vi "Write.Data.vi"(8 "error in (no error)":errorcluster, 10 "Values":dbl[](array[numeric]), 11 "Ref":refnum<data-value>) -> (0 "error out":errorcluster)   [LabVIEW 2015, in "Data Access Engine.lvlib" / "Data Access Engine.lvclass"]
uses:
  Data Access Engine.lvclass
  Data/Write/Write.lvclass
  Data/Write/Write.lvclass/Write.ctl
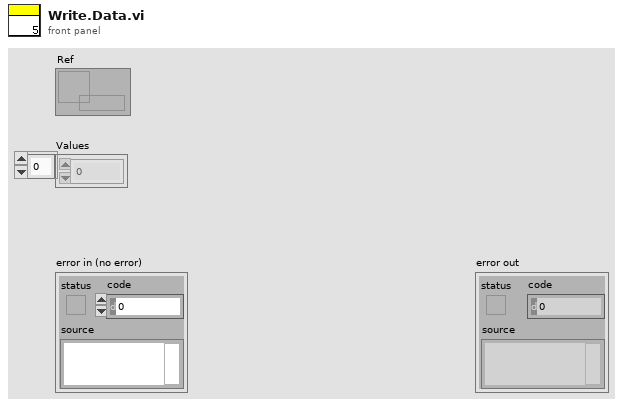
[diagram p1: front panel]
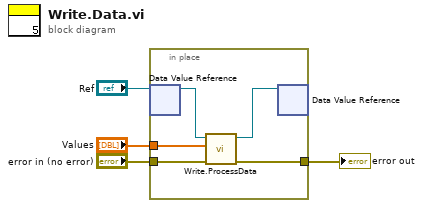
[diagram p0: block diagram]
diagram:
  n1 = in-place {
    in-place-border: "error in (no error)" -> [w9]
    in-place-border: [w8] -> w3
    in-place-border: "Values" -> [w5]
    n2 = in-place-dvr #1("Ref") -> (w7:refnum<class "Write.lvclass">)  [unwired: 1 out]
    n3 = call "Write.ProcessData.vi"("error in (no error)"=w9, "Values"=w5, "Write in"=w7) -> ("error out"=w8:errorcluster, "Write out"=w6:refnum<class "Write.lvclass">)  [unwired: 7 in]
    n4 = in-place-dvr #1(w6) -> ()  [unwired: 2 out]
  }
  "error out" <- w3
